vi "decimate true.vi"(10 "Boolean":bool=TRUE) -> (2 "every other true":bool)   [LabVIEW 2017]
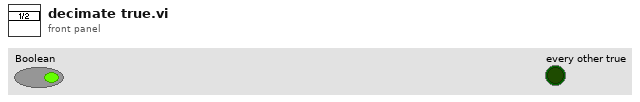
[diagram p1: front panel]
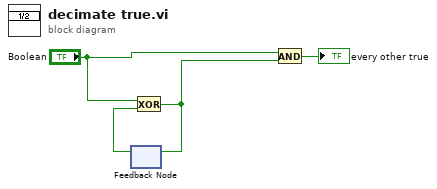
[diagram p0: block diagram]
diagram:
  n1 = feedback #1() -> (w4:bool)  [unwired: 1 in]
  n2 = Exclusive Or(1:w4, 2:"Boolean") -> (0:w3:bool)
  n3 = feedback-in #1(w3) -> ()
  n4 = And(x="Boolean", y=w3) -> (x .and. y?=→"every other true":bool)
